vi "convertRTPCInputBytes.vi"(6 "FullScale":dbl=24576.0, 7 "SCCM":dbl=500.0, 8 "RTPC Bytes":u8[](array[numeric])) -> (1 "Valve":u16, 2 "Pressure (SCCM)":dbl, 3 "Flow (SCCM)":dbl, 4 "Active Instance":u8, 5 "Status":bool[](array[boolean]))   [LabVIEW 2011]
uses:
  <vilib>/imath/engines/lvmath2/RunTimeEngine/NodeEndStatement/NIMS_NodeEndStatement_Output.vi
  <instcachedir>/0/NIMS_NodeEndStatement_Output_53EC0D466D134D7ABD903AC30B43404B.lvgen/NIMS_NodeEndStatement_Output_53EC0D466D134D7ABD903AC30B43404B_001.vi
  <vilib>/imath/engines/lvmath2/RunTimeEngine/ErrorHandling/NIMS_Finalize Error.vi
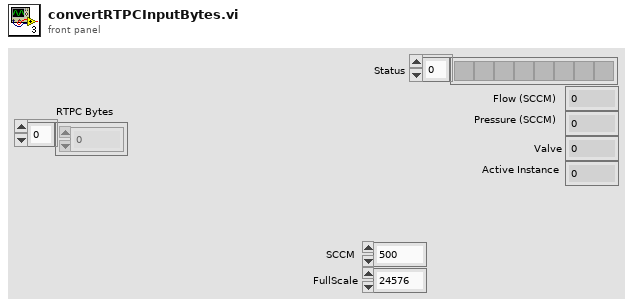
[diagram p1: front panel]
types:
  T1 = cluster{"[0]":u8, "[1]":u8, "[2]":u8, "[3]":u8, "[4]":u8, "[5]":u8, "[6]":u8, "[7]":u8}
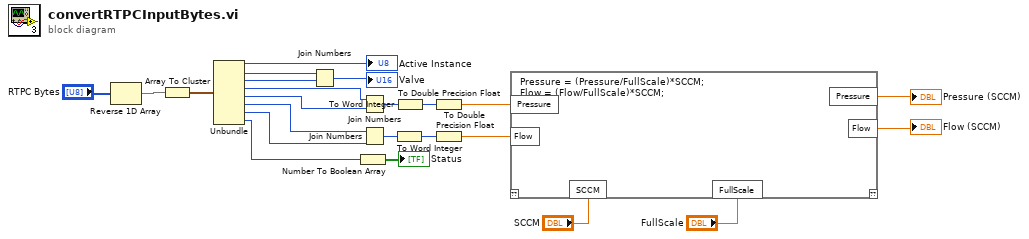
[diagram p0: block diagram]
diagram:
  n1 = Reverse 1D Array(array="RTPC Bytes") -> (reversed array=w17:u8[])
  n2 = Array To Cluster(array=w17) -> (cluster=w18:T1)
  n3 = Unbundle(w18) -> ("[0]"=→"Active Instance":u8, "[1]"=w6:u8, "[2]"=w7:u8, "[3]"=w12:u8, "[4]"=w13:u8, "[5]"=w14:u8, "[6]"=w15:u8, "[7]"=w16:u8)
  n4 = Join Numbers(hi=w6, lo=w7) -> ((hi.lo)=→"Valve":u16)
  n5 = Number To Boolean Array(number=w16) -> (Boolean array=→"Status":bool[])
  n6 = Join Numbers(hi=w12, lo=w13) -> ((hi.lo)=w8:u16)
  n7 = Join Numbers(hi=w14, lo=w15) -> ((hi.lo)=w9:u16)
  n8 = To Word Integer(number=w9) -> (16bit integer=w10:i16)
  n9 = To Word Integer(number=w8) -> (16bit integer=w11:i16)
  n10 = To Double Precision Float(number=w11) -> (double precision float=w22:dbl)
  n11 = To Double Precision Float(number=w10) -> (double precision float=w21:dbl)
  n12 = mathscript code="Pressure = (Pressure/FullScale)*SCCM;\nFlow = (Flow/FullScale)*SCCM;"("Flow"=w21, "Pressure"=w22, "SCCM"="SCCM", "FullScale"="FullScale") -> ("Flow"=→"Flow (SCCM)":dbl, "Pressure"=→"Pressure (SCCM)":dbl)  [unwired: 1 in, 1 out]
